vi "Main_MenuStrip_init.vi"(11 "MenuStrip":refnum<k24>) -> (2 "MenuItemStatusChange":refnum<user-event>, 3 "Menu out":refnum<class "MGI_MenuStrip.lvclass">)   [LabVIEW 2020]
doc: "Demonstrates the Menu Strip type. Run the VI to see the menu appear in the MenuStrip .NET control. Notice the \"File-> Default\"menu item that contains an icon as well as the \"File->Exit\" menu item contains a shortcut.\n\nClick summarys show up in the history array. Click the \"Add Item\" to add a dummy item to the MenuStrip's menu."
uses:
  System.Windows.Forms
  <userlib>/_MGI/Menu Building/MenuTypes/MenuStrip/MGI_MenuStrip.lvclass
  <userlib>/_MGI/Menu Building/MenuItemStatusChange/MGI_MenuItemStatusChange.lvclass
  <userlib>/_MGI/Menu Building/MenuItem/MenuSeparatorItem/MGI_MenuSeparatorItem.lvclass
  C:/Program Files (x86)/National Instruments/LabVIEW 2020/user.lib/_MGI/Menu Building/MenuItem/MGI_MenuItem.lvclass
  <userlib>/_MGI/Menu Building/MenuItem/MenuStripItem/MGI_MenuStripItem.lvclass
  <userlib>/_MGI/Menu Building/MenuItem/MenuItem.vi
  <userlib>/_MGI/Menu Building/MenuItem/MenuStripItem/MenuStripItem.vi
  <userlib>/_MGI/Menu Building/MenuTypes/MenuStrip/MenuStrip.vi
  <userlib>/_MGI/Menu Building/MenuItem/Write Sub-Menus.vi
  <userlib>/_MGI/Menu Building/MenuItem/MenuSeparatorItem/MenuSeparatorItem.vi
  <userlib>/_MGI/Menu Building/MenuItem/MGI_MenuItem.lvclass
  <userlib>/_MGI/Menu Building/MenuTypes/MGI_Menu.lvclass
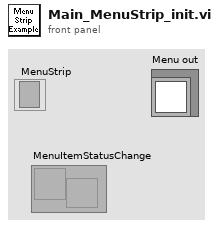
[diagram p1: front panel]
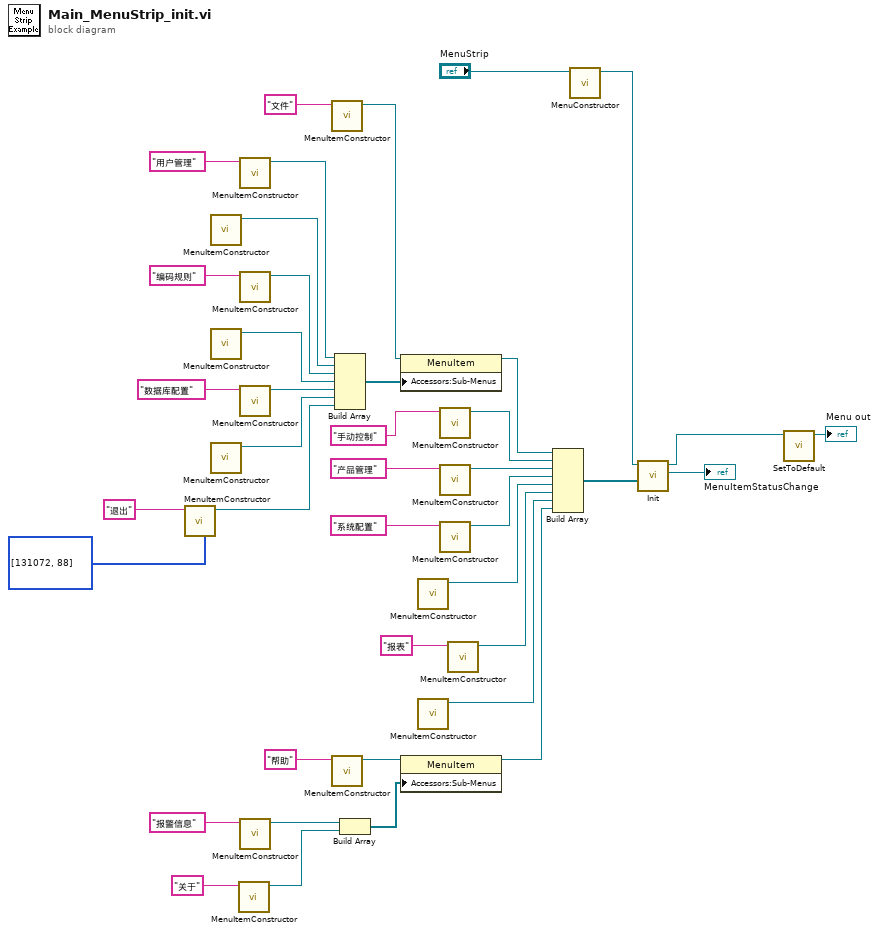
[diagram p0: block diagram]
diagram:
  w32 = i32[] [131072, 88] items=["None"=0, "LButton"=1, "RButton"=2, "Cancel"=3, "MButton"=4, "XButton1"=5, "XButton2"=6, "Back"=8, "Tab"=9, "LineFeed"=10, "Clear"=12, "Enter, Return"=13, "ShiftKey"=16, "ControlKey"=17, "Menu"=18, "Pause"=19, "CapsLock, Capital"=20, "HangulMode, HanguelMode, KanaMode"=21, "JunjaMode"=23, "FinalMode"=24, "KanjiMode, HanjaMode"=25, "Escape"=27, "IMEConvert"=28, "IMENonconvert"=29, "IMEAccept, IMEAceept"=30, "IMEModeChange"=31, "Space"=32, "Prior, PageUp"=33, "PageDown, Next"=34, "End"=35, "Home"=36, "Left"=37, "Up"=38, "Right"=39, "Down"=40, "Select"=41, "Print"=42, "Execute"=43, "Snapshot, PrintScreen"=44, "Insert"=45, "Delete"=46, "Help"=47, "D0"=48, "D1"=49, "D2"=50, "D3"=51, "D4"=52, "D5"=53, "D6"=54, "D7"=55, "D8"=56, "D9"=57, "A"=65, "B"=66, "C"=67, "D"=68, "E"=69, "F"=70, "G"=71, "H"=72, "I"=73, "J"=74, "K"=75, "L"=76, "M"=77, "N"=78, "O"=79, "P"=80, "Q"=81, "R"=82, "S"=83, "T"=84, "U"=85, "V"=86, "W"=87, "X"=88, "Y"=89, "Z"=90, "LWin"=91, "RWin"=92, "Apps"=93, "Sleep"=95, "NumPad0"=96, "NumPad1"=97, "NumPad2"=98, "NumPad3"=99, "NumPad4"=100, "NumPad5"=101, "NumPad6"=102, "NumPad7"=103, "NumPad8"=104, "NumPad9"=105, "Multiply"=106, "Add"=107, "Separator"=108, "Subtract"=109, "Decimal"=110, "Divide"=111, "F1"=112, "F2"=113, "F3"=114, "F4"=115, "F5"=116, "F6"=117, "F7"=118, "F8"=119, "F9"=120, "F10"=121, "F11"=122, "F12"=123, "F13"=124, "F14"=125, "F15"=126, "F16"=127, "F17"=128, "F18"=129, "F19"=130, "F20"=131, "F21"=132, "F22"=133, "F23"=134, "F24"=135, "NumLock"=144, "Scroll"=145, "LShiftKey"=160, "RShiftKey"=161, "LControlKey"=162, "RControlKey"=163, "LMenu"=164, "RMenu"=165, "BrowserBack"=166, "BrowserForward"=167, "BrowserRefresh"=168, "BrowserStop"=169, "BrowserSearch"=170, "BrowserFavorites"=171, "BrowserHome"=172, "VolumeMute"=173, "VolumeDown"=174, "VolumeUp"=175, "MediaNextTrack"=176, "MediaPreviousTrack"=177, "MediaStop"=178, "MediaPlayPause"=179, "LaunchMail"=180, "SelectMedia"=181, "LaunchApplication1"=182, "LaunchApplication2"=183, "OemSemicolon, Oem1"=186, "Oemplus"=187, "Oemcomma"=188, "OemMinus"=189, "OemPeriod"=190, "Oem2, OemQuestion"=191, "Oem3, Oemtilde"=192, "Oem4, OemOpenBrackets"=219, "OemPipe, Oem5"=220, "OemCloseBrackets, Oem6"=221, "OemQuotes, Oem7"=222, "Oem8"=223, "Oem102, OemBackslash"=226, "ProcessKey"=229, "Packet"=231, "Attn"=246, "Crsel"=247, "Exsel"=248, "EraseEof"=249, "Play"=250, "Zoom"=251, "NoName"=252, "Pa1"=253, "OemClear"=254, "KeyCode"=65535, "Shift"=65536, "Control"=131072, "Alt"=262144, "Modifiers"=-65536] ("Shortcut Keys")
  n1 = call-poly <userlib>:"MenuItemConstructor.vi"("Shortcut Keys"=w32, "Text"="退出") -> ("MenuStripItem"=w26:refnum<data-value>)  [unwired: 8 in, 1 out]
  n2 = call-poly <userlib>:"MenuItemConstructor.vi"() -> ("MenuSeparatorItem"=w6:refnum<data-value>)  [unwired: 10 in, 1 out]
  n3 = call-poly <userlib>:"MenuItemConstructor.vi"() -> ("MenuSeparatorItem"=w8:refnum<data-value>)  [unwired: 10 in, 1 out]
  n4 = call-poly <userlib>:"MenuItemConstructor.vi"() -> ("MenuSeparatorItem"=w34:refnum<data-value>)  [unwired: 10 in, 1 out]
  n5 = call-poly <userlib>:"MenuItemConstructor.vi"("Text"="关于") -> ("MenuItem"=w10:refnum<data-value>)  [unwired: 9 in, 1 out]
  n6 = call-poly <userlib>:"MenuItemConstructor.vi"("Text"="用户管理") -> ("MenuItem"=w5:refnum<data-value>)  [unwired: 9 in, 1 out]
  n7 = call-poly <userlib>:"MenuItemConstructor.vi"("Text"="编码规则") -> ("MenuItem"=w7:refnum<data-value>)  [unwired: 9 in, 1 out]
  n8 = call-poly <userlib>:"MenuItemConstructor.vi"("Text"="数据库配置") -> ("MenuItem"=w25:refnum<data-value>)  [unwired: 9 in, 1 out]
  n9 = call-poly <userlib>:"MenuItemConstructor.vi"("Text"="报警信息") -> ("MenuItem"=w11:refnum<data-value>)  [unwired: 9 in, 1 out]
  n10 = call-poly <userlib>:"MenuItemConstructor.vi"("Text"="文件") -> ("MenuItem"=w37:refnum<data-value>)  [unwired: 9 in, 1 out]
  n11 = call-poly <userlib>:"MenuItemConstructor.vi"("Text"="帮助") -> ("MenuItem"=w12:refnum<data-value>)  [unwired: 9 in, 1 out]
  n12 = Build Array(w5, w6, w7, w8, w25, w34, w26) -> (w38:refnum<data-value>[])
  n13 = Build Array(w11, w10) -> (w9:refnum<data-value>[])
  n14 = property class="MenuItem"(reference=w37, "Accessors:Sub-Menus"=w38) -> (reference out=w29:refnum<data-value>)  [unwired: 1 in, 1 out]
  n15 = property class="MenuItem"(reference=w12, "Accessors:Sub-Menus"=w9) -> (reference out=w2:refnum<data-value>)  [unwired: 1 in, 1 out]
  n16 = call-poly <userlib>:"MenuItemConstructor.vi"() -> ("MenuSeparatorItem"=w13:refnum<data-value>)  [unwired: 10 in, 1 out]
  n17 = call-poly <userlib>:"MenuItemConstructor.vi"() -> ("MenuSeparatorItem"=w3:refnum<data-value>)  [unwired: 10 in, 1 out]
  n18 = call-poly <userlib>:"MenuItemConstructor.vi"("Text"="手动控制") -> ("MenuItem"=w16:refnum<data-value>)  [unwired: 9 in, 1 out]
  n19 = call-poly <userlib>:"MenuItemConstructor.vi"("Text"="产品管理") -> ("MenuItem"=w15:refnum<data-value>)  [unwired: 9 in, 1 out]
  n20 = call-poly <userlib>:"MenuItemConstructor.vi"("Text"="系统配置") -> ("MenuItem"=w14:refnum<data-value>)  [unwired: 9 in, 1 out]
  n21 = call-poly <userlib>:"MenuItemConstructor.vi"("Text"="报表") -> ("MenuItem"=w4:refnum<data-value>)  [unwired: 9 in, 1 out]
  n22 = Build Array(w29, w16, w15, w14, w13, w4, w3, w2) -> (w39:refnum<data-value>[])
  n23 = call-poly <userlib>:"MenuConstructor.vi"("MenuStrip"="MenuStrip") -> ("MenuStrip out"=w30:refnum<class "MGI_MenuStrip.lvclass">)  [unwired: 9 in, 1 out]
  n24 = call-dynamic "Init.vi"("Menu Items"=w39, "Menu in"=w30) -> ("MenuItemStatusChange"=→"MenuItemStatusChange":refnum<user-event>, "Menu out"=w40:refnum<class "MGI_MenuStrip.lvclass">)  [unwired: 7 in, 1 out]
  n25 = call-dynamic "SetToDefault.vi"("Menu in"=w40) -> ("Menu out"=→"Menu out":refnum<class "MGI_MenuStrip.lvclass">)  [unwired: 9 in, 1 out]
